vi "hse-configuration_ParseConfigSource.vi"(8 "error in (no error)":errorcluster, 10 "Config Source":variant, 11 "hse-config-ini in":refnum<class "hse-config-ini.lvclass">) -> (0 "error out":errorcluster, 3 "hse-config-ini out":refnum<class "hse-config-ini.lvclass">)   [LabVIEW 2014, in "hse-config-ini.lvclass"]
doc: "Reads the contents of the configuration file and keeps them in memory"
uses:
  hse-config-ini.lvclass
  hse-config-ini_ConfigData.ctl
  hse-configuration.lvclass/hse-configuration.ctl
  hse-configuration_ReadDataDirectory.vi
  hse-configuration_WriteDataDirectory.vi
  <vilib>/Utility/config.llb/Read Key (String).vi
  <vilib>/Utility/config.llb/NI_LVConfig.lvlib
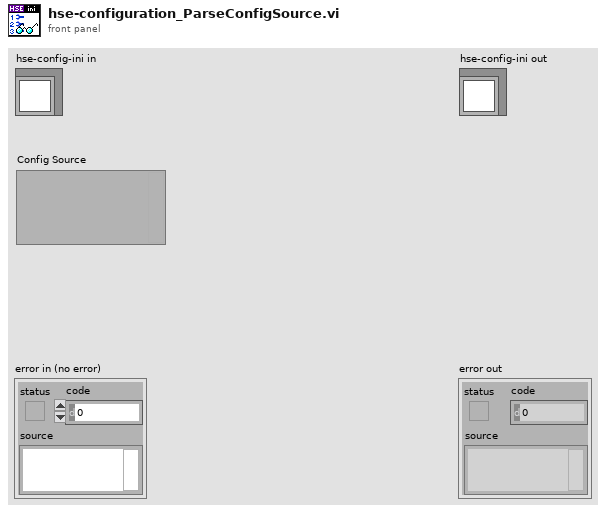
[diagram p1: front panel]
types:
  T1 = typedef "hse-config-ini.lvclass/hse-config-ini_ConfigData.ctl" = cluster{"Path to .ini file":path}
  T2 = typedef "NI_LVConfig.lvlib/Config Data RefNum.ctl" = refnum<k1>
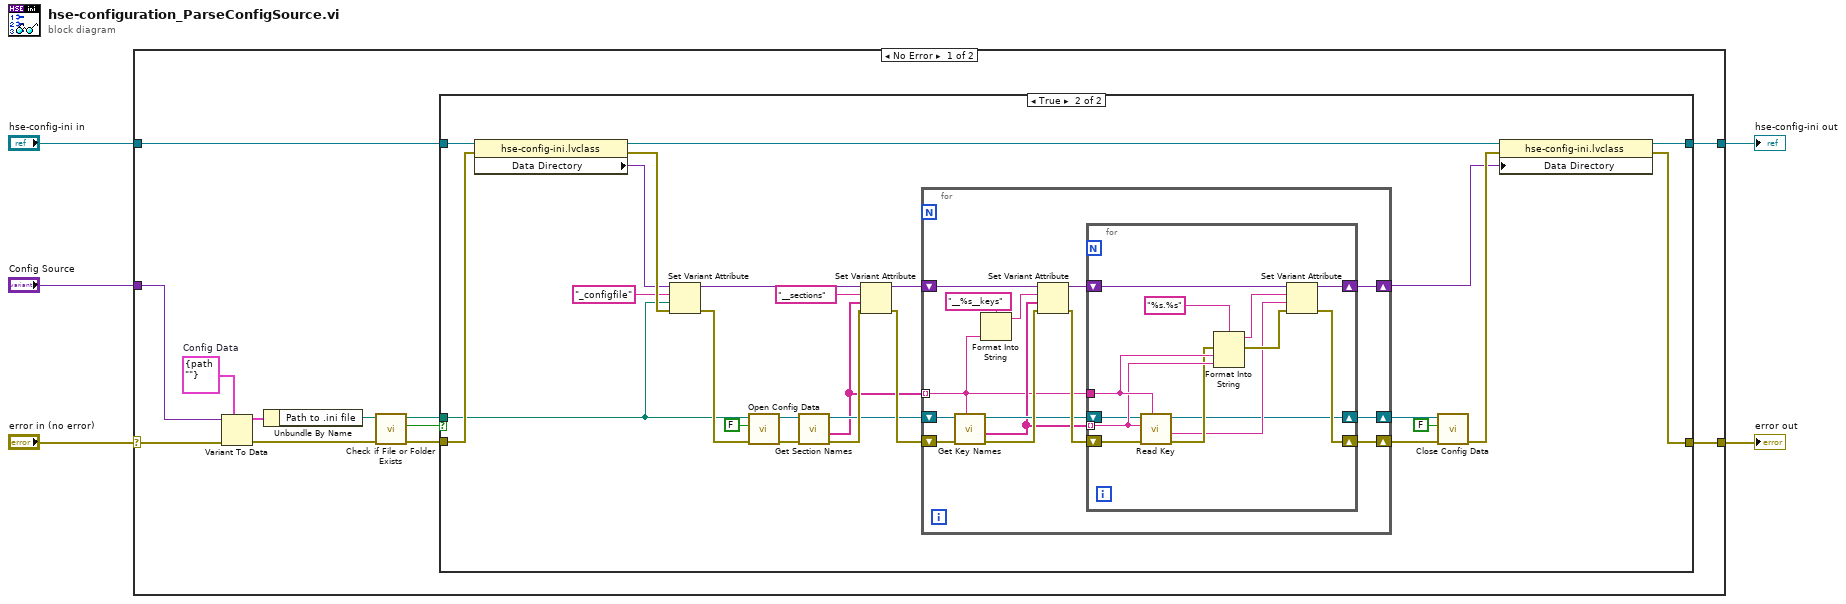
[diagram p0: block diagram]
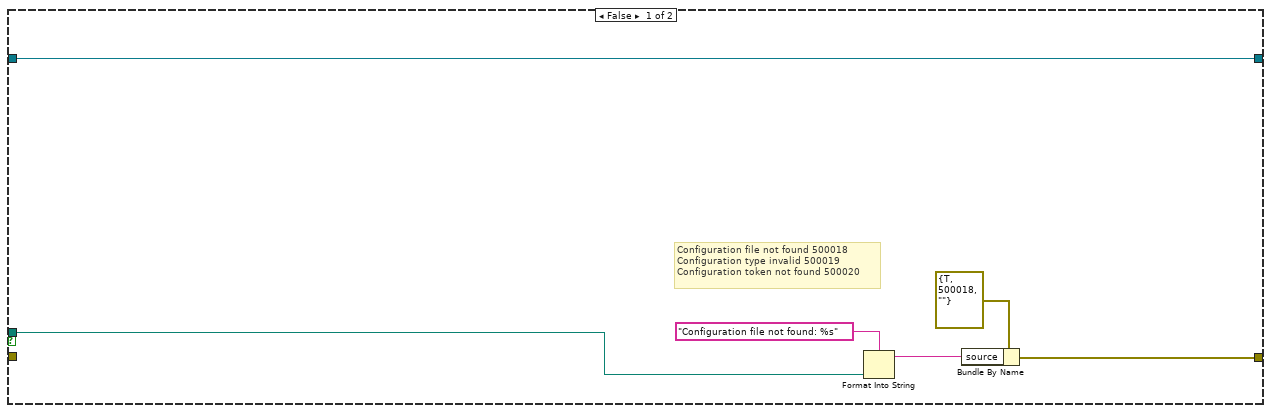
[diagram p2: hidden frame]
diagram:
  n1 = case shown="No Error" "error in (no error)" {
    selector: "error in (no error)" -> [w15 w77]
    tunnel: [w12 w77] -> w4
    tunnel: "hse-config-ini in" -> [w14 w76]
    tunnel: [w13 w76] -> w2
    tunnel: "Config Source" -> [w17 _]
    frame No Error {
      w16 = T1 {"Path to .ini file"=path ""}  # Config Data
      n2 = Variant To Data(error in=w15, type=w16, Variant=w17) -> (data=w11:T1, error out=w7:errorcluster)
      n3 = Unbundle By Name(w11) -> ("Path to .ini file"=w10:path)
      n4 = call <vilib>:"Check if File or Folder Exists.vi"("error in (no error)"=w7, "path"=w10) -> ("error out"=w6:errorcluster, "file or folder exists?"=w8:bool, "dup path"=w9:path)  [unwired: 7 in]
      n5 = case shown="True" w8 {
        tunnel: w14 -> [w23 w43]
        tunnel: [w23 w41] -> w13
        tunnel: [w18 w40] -> w12
        tunnel: w9 -> [w22 w29]
        tunnel: w6 -> [_ w31]
        frame False {
          # "Configuration file not found\t500018\nConfiguration type invalid\t500019\nConfiguration token not found\t500020"
          n6 = Format Into String(format string="Configuration file not found: %s", w22) -> (resulting string=w20:string)  [unwired: 2 in, 1 out]
          n7 = Bundle By Name(cluster=errorcluster {"status"=TRUE, "code"=500018, "source"=""} ("error in (no error)"), "source"=w20) -> (w18:errorcluster)
        }
        frame True {
          n8 = property class="hse-config-ini.lvclass"(reference=w43, error in=w31) -> (reference out=w42:refnum<class "hse-config-ini.lvclass">, error out=w33:errorcluster, "Data Directory"=w28:variant)
          n9 = Set Variant Attribute(Variant=w28, name="_configfile", value=w29, error in=w33) -> (Variant out=w25:variant, error out=w30:errorcluster)  [unwired: 1 out]
          n10 = call <vilib>:"Open Config Data.vi"("error in (no error)"=w30, "create file if necessary (T)"=FALSE, "configuration file path"=w29) -> ("error out"=w44:errorcluster, "refnum"=w45:T2)  [unwired: 6 in, 1 out]
          n11 = call <vilib>:"Get Section Names.vi"("error in (no error)"=w44, "refnum"=w45) -> ("error out"=w48:errorcluster, "section names"=w24:string[], "refnum out"=w39:T2)  [unwired: 7 in]
          n12 = Set Variant Attribute(Variant=w25, name="__sections", value=w24, error in=w48) -> (Variant out=w26:variant, error out=w47:errorcluster)  [unwired: 1 out]
          n13 = for {
            shift-right: [w57] -> w37
            shift-left: w47 -> [w58]
            tunnel: w24 -> [w49] mode=indexing
            shift-right: [w56] -> w34
            shift-left: w26 -> [w54]
            shift-right: [w55] -> w38
            shift-left: w39 -> [w60]
            n14 = call <vilib>:"Get Key Names.vi"("section"=w49, "error in (no error)"=w58, "refnum"=w60) -> ("error out"=w62:errorcluster, "key names"=w50:string[], "refnum out"=w59:T2)  [unwired: 5 in, 1 out]
            n15 = Format Into String(format string="__%s__keys" ("name"), w49) -> (resulting string=w51:string)  [unwired: 2 in, 1 out]
            n16 = Set Variant Attribute(Variant=w54, name=w51, value=w50, error in=w62) -> (Variant out=w53:variant, error out=w61:errorcluster)  [unwired: 1 out]
            n17 = for {
              shift-right: [w66] -> w57
              shift-left: w61 -> [w75]
              tunnel: w49 -> [w70]
              tunnel: w50 -> [w69] mode=indexing
              shift-right: [w73] -> w56
              shift-left: w53 -> [w74]
              shift-right: [w63] -> w55
              shift-left: w59 -> [w65]
              n18 = call-poly <vilib>:"Read Key.vi"("section"=w70, "error in (no error)"=w75, "key"=w69, "refnum"=w65) -> ("error out"=w67:errorcluster, "value"=w64:string, "refnum out"=w63:T2)  [unwired: 4 in, 1 out]
              n19 = Format Into String(format string="%s.%s", error in=w67, w70, w69) -> (resulting string=w71:string, error out=w68:errorcluster)  [unwired: 1 in]
              n20 = Set Variant Attribute(Variant=w74, name=w71, value=w64, error in=w68) -> (Variant out=w73:variant, error out=w66:errorcluster)  [unwired: 1 out]
            }
          }
          n21 = call <vilib>:"Close Config Data.vi"("error in (no error)"=w37, "write file if changed (T)"=FALSE, "refnum"=w38) -> ("error out"=w36:errorcluster)  [unwired: 7 in, 1 out]
          n22 = property class="hse-config-ini.lvclass"(reference=w42, error in=w36, "Data Directory"=w34) -> (reference out=w41:refnum<class "hse-config-ini.lvclass">, error out=w40:errorcluster)
        }
      }
    }
    frame Error {
    }
  }
  "error out" <- w4
  "hse-config-ini out" <- w2
